vi "Create Unique Notifier.vi"(8 "error in":errorcluster, 9 "DAQ task to send":refnum<k21>, 10 "Send? (T)":bool, 11 "Device Ref":T1 format="%.0x") -> (0 "error out":errorcluster, 2 "DAQ task received":refnum<k21>, 3 "Device Ref dup":T1 format="%.0x", 5 "created new?":bool)   [LabVIEW 2011, in "PXIe-433x Custom Device.lvlib"]
uses:
  PXIe-433x Custom Device.lvlib
  <vilib>/NI Veristand/Custom Device API/Custom Device Item Ref.ctl
  <vilib>/NI Veristand/Custom Device API/Custom Device API.lvlib
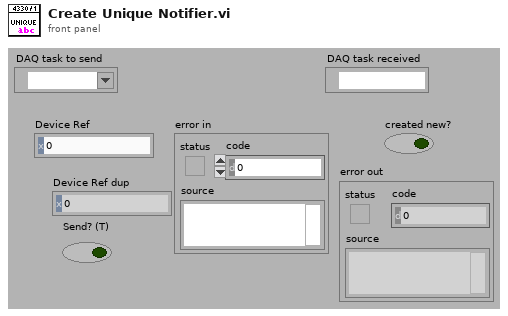
[diagram p1: front panel]
types:
  T1 = typedef "Custom Device API.lvlib/Custom Device Item Ref.ctl" = u64
  T2 = typedef "Custom Device API.lvlib/Custom Device Item Info.ctl" = cluster{"Name":string, "Is Channel":bool, "GUID":string}
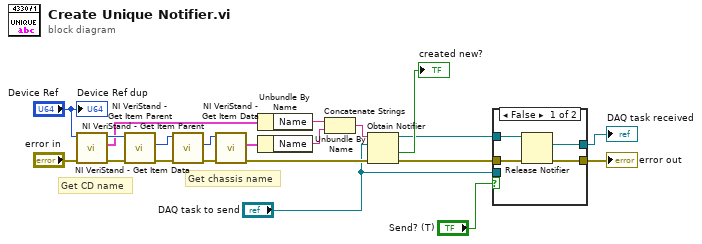
[diagram p0: block diagram]
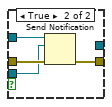
[diagram p2: hidden frame]
diagram:
  # "Get chassis name"
  # "Get CD name"
  n1 = call <vilib>:"NI VeriStand - Get Item Data.vi"("error in (no error)"="error in", "Item Ref in"="Device Ref") -> ("error out"=w10:errorcluster, "Item Info"=w9:T2, "Item Ref out"=w11:T1)  [unwired: 6 in, 1 out]
  n2 = call <vilib>:"NI VeriStand - Get Item Parent.vi"("error in (no error)"=w10, "Item Ref in"=w11) -> ("error out"=w12:errorcluster, "Parent Ref"=w13:T1)  [unwired: 6 in, 2 out]
  n3 = call <vilib>:"NI VeriStand - Get Item Parent.vi"("error in (no error)"=w12, "Item Ref in"=w13) -> ("error out"=w14:errorcluster, "Parent Ref"=w15:T1)  [unwired: 6 in, 2 out]
  n4 = call <vilib>:"NI VeriStand - Get Item Data.vi"("error in (no error)"=w14, "Item Ref in"=w15) -> ("error out"=w20:errorcluster, "Item Info"=w16:T2)  [unwired: 6 in, 2 out]
  n5 = Unbundle By Name(w9) -> ("Name"=w18:string)
  n6 = Unbundle By Name(w16) -> ("Name"=w17:string)
  n7 = Concatenate Strings(w18, w17) -> (w19:string)
  n8 = Obtain Notifier(name (unnamed)=w19, notification data type="DAQ task to send", error in (no error)=w20) -> (notifier out=w3:refnum<notifier>, created new?=→"created new?":bool, error out=w6:errorcluster)  [unwired: 1 in]
  n9 = case shown="False" "Send? (T)" {
    tunnel: w6 -> [w24 w29]
    tunnel: [w25 w28] -> w5
    tunnel: w3 -> [w23 w27]
    tunnel: "DAQ task to send" -> [_ w26]
    tunnel: [w22 _] -> w1
    frame False {
      n10 = Release Notifier(notifier=w23, error in (no error)=w24) -> (last notification=w22:refnum<k21>, error out=w25:errorcluster)  [unwired: 1 in, 1 out]
    }
    frame True {
      n11 = Send Notification(notification=w26, notifier=w27, error in (no error)=w29) -> (error out=w28:errorcluster)  [unwired: 1 out]
    }
  }
  "error out" <- w5
  "DAQ task received" <- w1
  "Device Ref dup" <- "Device Ref"
